vi "Write Column Index.vi"(10 "Column Index":i32, 11 "Change Column Header in":refnum<class "Change Column Header.lvclass">) -> (3 "Change Column Header out":refnum<class "Change Column Header.lvclass">)   [LabVIEW 2016, in "Assert API Components.lvlib" / "Assert Display.lvlib" / "Main Display.lvlib" / "Change Column Header.lvclass"]
uses:
  Change Column Header.lvclass
  Change Column Header.lvclass/Change Column Header.ctl
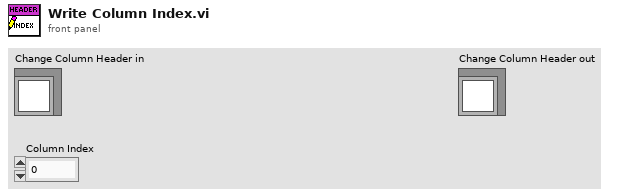
[diagram p1: front panel]
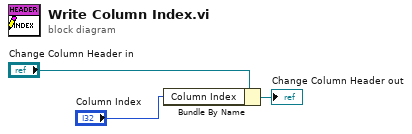
[diagram p0: block diagram]
diagram:
  n1 = Bundle By Name(cluster="Change Column Header in", "Column Index"="Column Index") -> (→"Change Column Header out":refnum<class "Change Column Header.lvclass">)
